vi "Move Part.vi"(8 "error in (no error)":errorcluster, 10 "XRay Table.lvclass":refnum<class "XRay Table.lvclass">, 11 "XRay Part Sample in":refnum<class "XRay Part Sample.lvclass">) -> (0 "error out":errorcluster, 3 "XRay Part Sample out":refnum<class "XRay Part Sample.lvclass">)   [LabVIEW 2026, in "XRay Part Sample.lvclass"]
uses:
  XRay Part Sample.lvclass
  XRay Table/XRay Table.lvclass
  XRay Part Sample.lvclass/XRay Part Sample.ctl
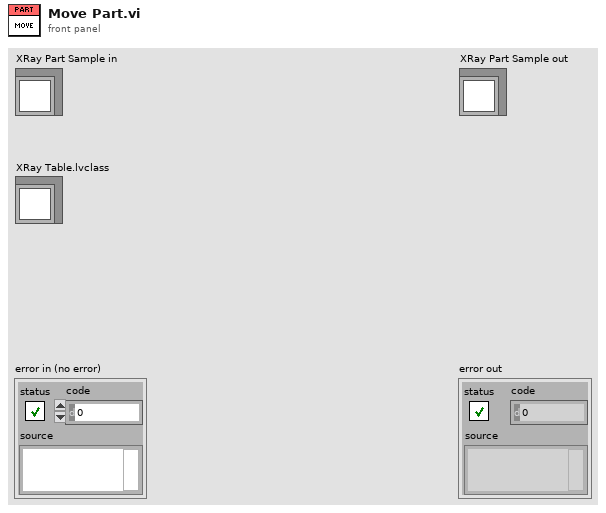
[diagram p1: front panel]
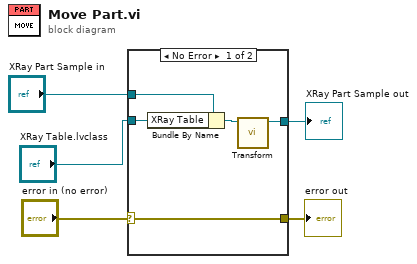
[diagram p0: block diagram]
diagram:
  n1 = case shown="No Error" "error in (no error)" {
    selector: "error in (no error)" -> [w10 w11]
    tunnel: [w10 w11] -> w4
    tunnel: [w8 w12] -> w2
    tunnel: "XRay Part Sample in" -> [w6 w12]
    tunnel: "XRay Table.lvclass" -> [w9 _]
    frame No Error {
      n2 = Bundle By Name(cluster=w6, "XRay Table"=w9) -> (w7:refnum<class "XRay Part Sample.lvclass">)
      n3 = call-dynamic "Transform.vi"("XRay Part Sample in"=w7) -> ("XRay Part Sample out"=w8:refnum<class "XRay Part Sample.lvclass">)  [unwired: 9 in, 1 out]
    }
    frame Error {
    }
  }
  "error out" <- w4
  "XRay Part Sample out" <- w2
